vi "GenerateFilepathLA.vi"(4 "Auto Date folder":bool, 5 "Filename":string="Spectrometer_", 6 "base path":path=path "M:/Oceanoptics/TDMS test") -> (0 "operation (0:open)":T1(ring), 1 "file path":path=path "M:/Oceanoptics/TDMS test/Spectrometer_test213.tdms", 2 "Folder Path":path)   [LabVIEW 2017]
uses:
  <vilib>/regexp/Match Regular Expression.xnode
panel:
  out "Month":string
  out "Year":string
  out "Day":string
  out "date string":string
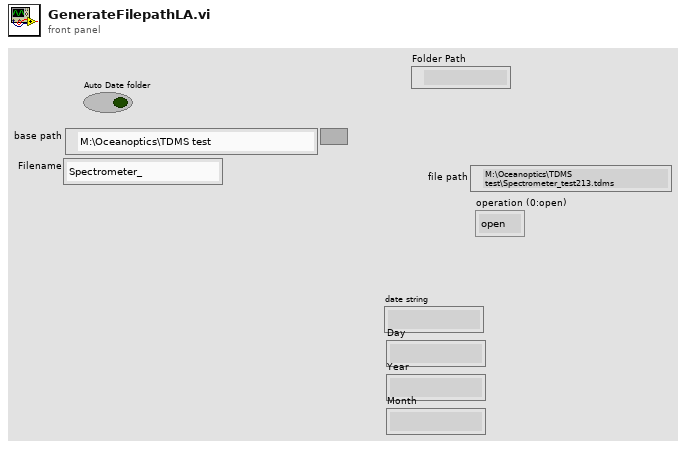
[diagram p1: front panel]
types:
  T1 = enum16{"open", "open or create", "create or replace", "create", "open (read-only)"}
  T2 = enum16{"Left Button", "Center Button", "Right Button", "Window Close"}
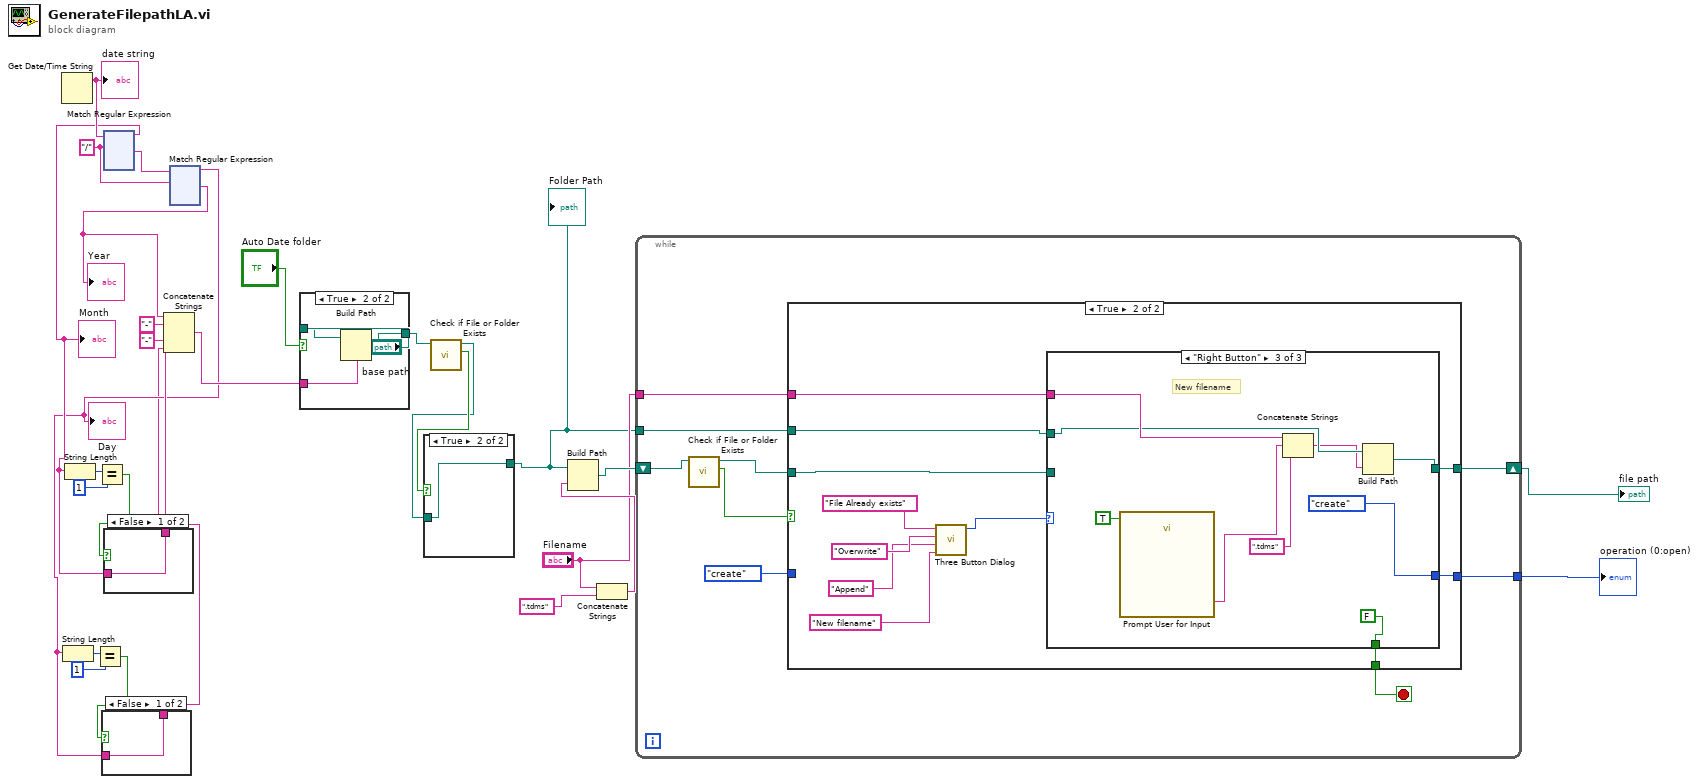
[diagram p0: block diagram]
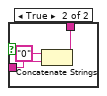
[diagram p2: hidden frame]
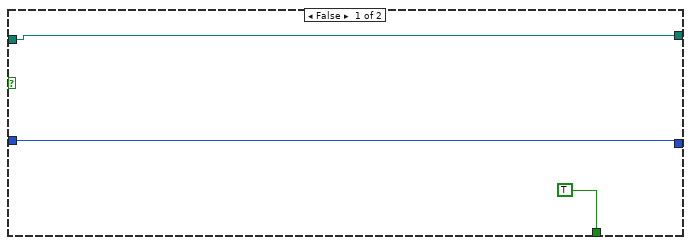
[diagram p3: hidden frame]
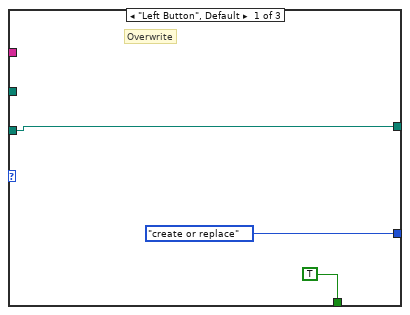
[diagram p4: hidden frame]
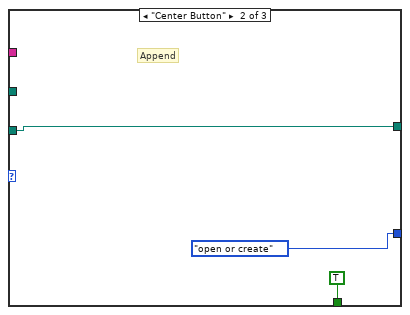
[diagram p5: hidden frame]
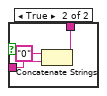
[diagram p6: hidden frame]
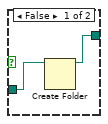
[diagram p7: hidden frame]
diagram:
  w26 = "/" ("regular expression")
  n1 = Get Date/Time String() -> (date string=w28:string)  [unwired: 3 in, 1 out]
  "date string" <- w28
  n2 = xnode "Match Regular Expression"("input string"=w28, "regular expression"=w26) -> ("before match"=w13:string, "after match"=w27:string)  [unwired: 4 in, 3 out]
  "Month" <- w13
  n3 = String Length(string=w13) -> (length=w16:i32)
  n4 = Equal?(x=w16, y=1) -> (x = y?=w14:bool)
  n5 = case shown="False" w14 {
    tunnel: w13 -> [w30 w33]
    tunnel: [w30 w31] -> w12
    frame False {
    }
    frame True {
      n6 = Concatenate Strings("0" ("string"), w33) -> (w31:string)
    }
  }
  n7 = xnode "Match Regular Expression"("input string"=w27, "regular expression"=w26) -> ("before match"=w3:string, "after match"=w17:string)  [unwired: 4 in, 3 out]
  "Day" <- w3
  "Year" <- w17
  n8 = String Length(string=w3) -> (length=w4:i32)
  n9 = Equal?(x=w4, y=1) -> (x = y?=w6:bool)
  n10 = case shown="False" w6 {
    tunnel: w3 -> [w34 w37]
    tunnel: [w34 w35] -> w2
    frame False {
    }
    frame True {
      n11 = Concatenate Strings("0" ("string"), w37) -> (w35:string)
    }
  }
  n12 = Concatenate Strings(w17, "-" ("string"), w12, "-" ("string"), w2) -> (w21:string)
  n13 = case shown="True" "Auto Date folder" {
    tunnel: "base path" -> [w38 w41]
    tunnel: [w38 w39] -> w20
    tunnel: w21 -> [_ w40]
    frame False {
    }
    frame True {
      n14 = Build Path(base path=w41, name or relative path=w40) -> (appended path=w39:path)
    }
  }
  n15 = call <vilib>:"Check if File or Folder Exists.vi"("path"=w20) -> ("file or folder exists?"=w19:bool, "dup path"=w18:path)  [unwired: 8 in, 1 out]
  n16 = case shown="True" w19 {
    tunnel: w18 -> [w43 w44]
    tunnel: [w42 w44] -> w9
    frame False {
      n17 = Create Folder(path (use dialog)=w43) -> (created path=w42:path)  [unwired: 2 in, 2 out]
    }
    frame True {
    }
  }
  "Folder Path" <- w9
  n18 = Concatenate Strings("Filename", ".tdms" ("string")) -> (w29:string)
  n19 = Build Path(base path=w9, name or relative path=w29) -> (appended path=w11:path)
  n20 = while {
    tunnel: "Filename" -> [w48]
    tunnel: w9 -> [w47]
    shift-right: [w46] -> w8
    shift-left: w11 -> [w53]
    tunnel: [w45] -> w7
    stop <- w49 stop-if-true
    n21 = call <vilib>:"Check if File or Folder Exists.vi"("path"=w53) -> ("file or folder exists?"=w52:bool, "dup path"=w51:path)  [unwired: 8 in, 1 out]
    n22 = case shown="True" w52 {
      tunnel: w51 -> [w54 w62]
      tunnel: w48 -> [_ w61]
      tunnel: [w56 w60] -> w45
      tunnel: T1."create" ("operation (0:open)") -> [w56 _]
      tunnel: [TRUE w59] -> w49
      tunnel: w47 -> [_ w58]
      tunnel: [w54 w57] -> w46
      frame False {
      }
      frame True {
        n23 = call <vilib>:"Three Button Dialog.vi"("Right Button Text (\"Cancel\")"="New filename" ("Right Button Text (\"Cancel\")"), "Center Button Text (\"No\")"="Append" ("Center Button Text (\"No\")"), "Left Button Text (\"Yes\")"="Overwrite" ("Left Button Text (\"Yes\")"), "message"="File Already exists") -> ("Which Button?"=w63:T2)  [unwired: 7 in]
        n24 = case shown="\"Right Button\"" w63 {
          tunnel: w62 -> [w68 w71 _]
          tunnel: w61 -> [_ _ w77]
          tunnel: [T1."create or replace" ("operation (0:open)") T1."open or create" ("operation (0:open)") T1."create" ("operation (0:open)")] -> w60
          tunnel: [TRUE TRUE FALSE] -> w59
          tunnel: w58 -> [_ _ w76]
          tunnel: [w68 w71 w74] -> w57
          frame "Left Button", Default {
            # "Overwrite"
          }
          frame "Center Button" {
            # "Append"
          }
          frame "Right Button" {
            # "New filename"
            n25 = call "Prompt User for Input"("Enable"=TRUE) -> ("Filename Append"=w78:string)  [unwired: 16 in, 2 out]
            n26 = Concatenate Strings(w77, w78, ".tdms" ("string")) -> (w75:string)
            n27 = Build Path(base path=w76, name or relative path=w75) -> (appended path=w74:path)
          }
        }
      }
    }
  }
  "file path" <- w8
  "operation (0:open)" <- w7
